vi "Skip Next.vi"(8 "error in (no error)":errorcluster, 11 "LUnit Test Suite In":refnum<class "LUnit Test Suite.lvclass">) -> (0 "error out":errorcluster, 3 "LUnit Test Suite Out":refnum<class "LUnit Test Suite.lvclass">)   [LabVIEW 2020, in "LUnit Test Suite.lvclass"]
uses:
  LUnit Test Suite.lvclass
  LUnit Test Suite.lvclass/LUnit Test Suite.ctl
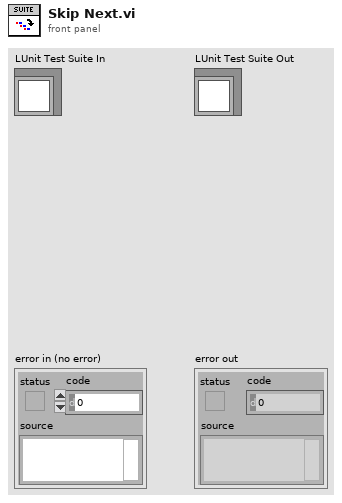
[diagram p1: front panel]
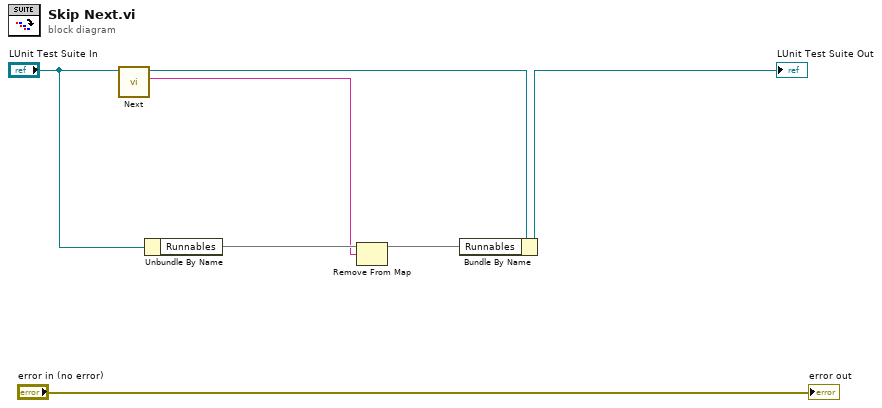
[diagram p0: block diagram]
diagram:
  n1 = call-dynamic "Next.vi"("LUnit Test Suite In"="LUnit Test Suite In") -> ("Name"=w4:string, "LUnit Test Suite Out"=w7:refnum<class "LUnit Test Suite.lvclass">)  [unwired: 7 in, 2 out]
  n2 = Unbundle By Name("LUnit Test Suite In") -> ("Runnables"=w5:map{string, refnum<class "Runnable.lvclass">})
  n3 = Remove From Map(10:w4, 11:w5) -> (3:w1:map{string, refnum<class "Runnable.lvclass">})  [unwired: 2 out]
  n4 = Bundle By Name(cluster=w7, "Runnables"=w1) -> (→"LUnit Test Suite Out":refnum<class "LUnit Test Suite.lvclass">)
  "error out" <- "error in (no error)"
